vi "Display_FGV.vi"(7 "Display_mods":T1, 8 "error in":errorcluster, 11 "variant":variant) -> (0 "error out":errorcluster, 3 "Base":picture)   [LabVIEW 2017]
uses:
  Display_mods.ctl
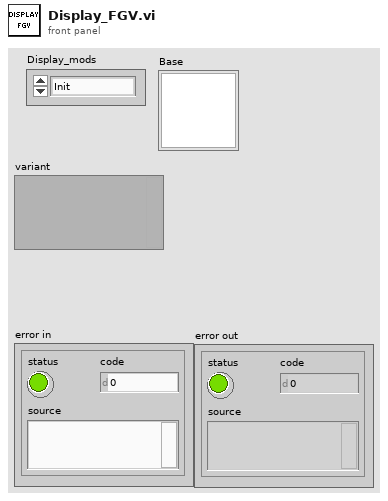
[diagram p1: front panel]
types:
  T1 = typedef "Display_mods.ctl" = enum16{"Init", "GetBase", "DrawAster", "Clear", "Close"}
  T2 = cluster{"rect":cluster{"left":i16, "top":i16, "right":i16, "bottom":i16}, "Fill":bool}
  T3 = cluster{"left":i16, "top":i16, "right":i16, "bottom":i16}
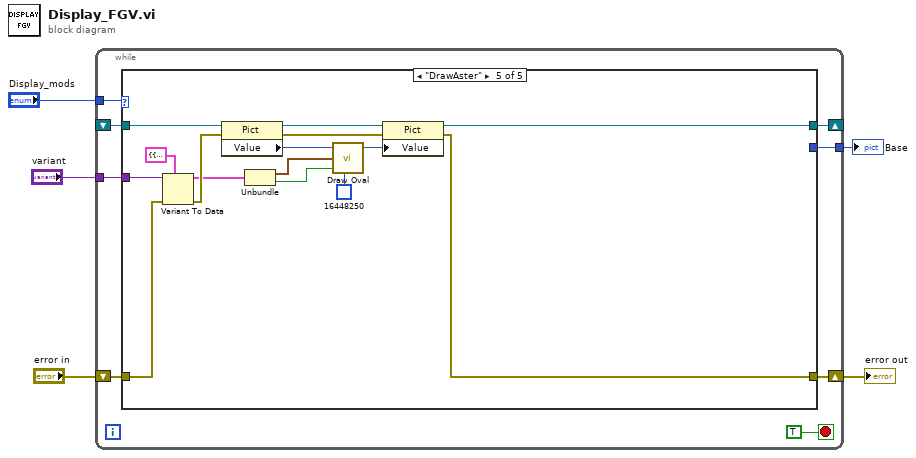
[diagram p0: block diagram]
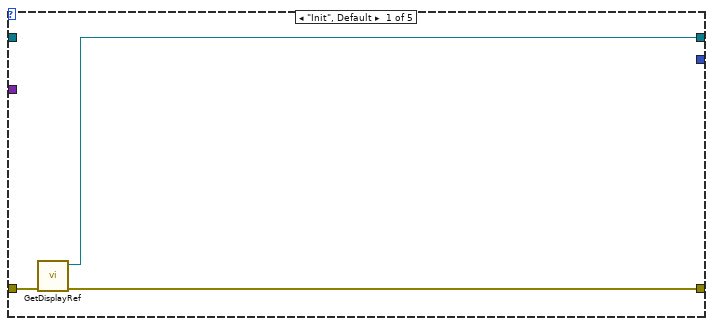
[diagram p2: hidden frame]
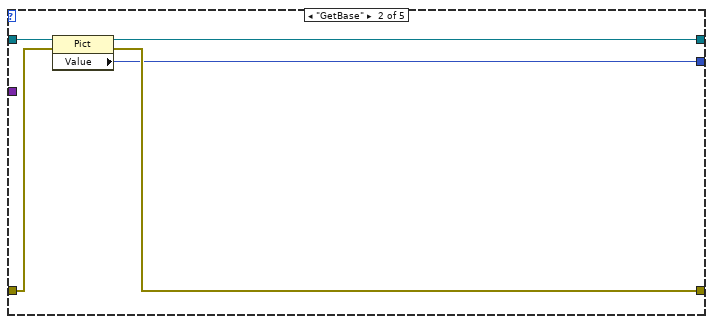
[diagram p3: hidden frame]
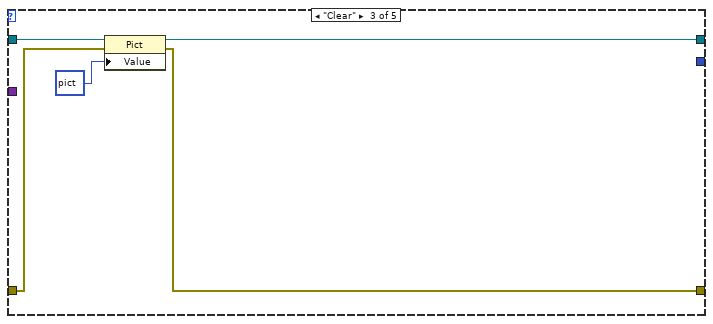
[diagram p4: hidden frame]
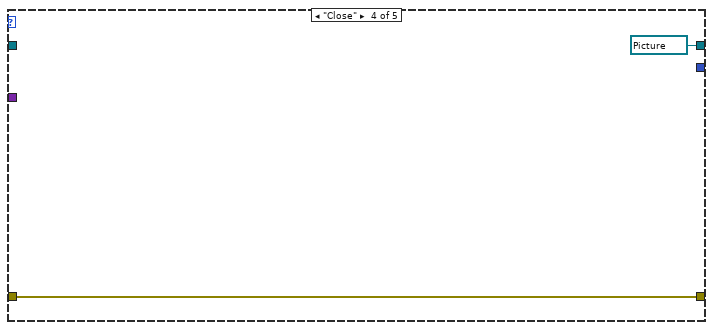
[diagram p5: hidden frame]
diagram:
  n1 = while {
    shift-right: [w10] -> w4
    shift-left: "error in" -> [w13]
    tunnel: "Display_mods" -> [w11]
    shift-right: [w8] -> _
    shift-left: _ -> [w9]
    tunnel: [w7] -> w2
    tunnel: "variant" -> [w6]
    stop <- TRUE stop-if-true
    n2 = case shown="\"DrawAster\"" w11 {
      tunnel: w13 -> [w16 w21 w22 w27 w40]
      tunnel: [w14 w19 w23 w27 w43] -> w10
      tunnel: w9 -> [_ w20 w26 _ w38]
      tunnel: [w15 w18 w25 refnum<vi> refnum ("Picture out") w42] -> w8
      tunnel: [_ w17 _ _ _] -> w7
      tunnel: w6 -> [_ _ _ _ w41]
      frame "Init", Default {
        n3 = call "GetDisplayRef.vi"("error in"=w16) -> ("error out"=w14:errorcluster, "Picture out"=w15:refnum<vi>)  [unwired: 9 in]
      }
      frame "GetBase" {
        n4 = property class="Pict"(reference=w20, error in=w21) -> (reference out=w18:refnum<vi>, error out=w19:errorcluster, "Value"=w17:picture)
      }
      frame "Clear" {
        n5 = property class="Pict"(reference=w26, error in=w22, "Value"=picture data[5B]) -> (reference out=w25:refnum<vi>, error out=w23:errorcluster)
      }
      frame "Close" {
      }
      frame "DrawAster" {
        n6 = Variant To Data(error in=w40, type=T2 {"rect"={"left"=0, "top"=0, "right"=0, "bottom"=0}, "Fill"=FALSE} ("output cluster"), Variant=w41) -> (data=w35:T2, error out=w37:errorcluster)
        n7 = property class="Pict"(reference=w38, error in=w37) -> (reference out=w29:refnum<vi>, error out=w30:errorcluster, "Value"=w34:picture)
        n8 = Unbundle(w35) -> ("rect"=w32:T3, "Fill"=w33:bool)
        n9 = call <vilib>:"Draw Oval.vi"("picture"=w34, "rect"=w32, "fill?(F)"=w33, "color(black)"=u32 16448250) -> ("new picture"=w31:picture)  [unwired: 5 in]
        n10 = property class="Pict"(reference=w29, error in=w30, "Value"=w31) -> (reference out=w42:refnum<vi>, error out=w43:errorcluster)
      }
    }
  }
  "error out" <- w4
  "Base" <- w2
